vi "Launch Settings Dialog.vi"(8 "error in (no error)":errorcluster, 11 "Controller in":refnum<class "Controller.lvclass">) -> (0 "error out":errorcluster, 3 "Controller out":refnum<class "Controller.lvclass">)   [LabVIEW 2026, in "Controller Actor.lvlib" / "Controller.lvclass"]
uses:
  Controller.lvclass
  C:/Program Files/National Instruments/LabVIEW 2026/vi.lib/ActorFramework/Actor/Actor.lvclass
  Controller.lvclass/Controller.ctl
  <vilib>/ActorFramework/Actor/Actor.lvclass/Actor.ctl
  <vilib>/ActorFramework/Message Enqueuer/Message Enqueuer.lvclass/Message Enqueuer.ctl
  <vilib>/ActorFramework/Message Enqueuer/Init from Existing Queue.vi
  configuration/Configuration.lvclass
  <vilib>/ActorFramework/Message Enqueuer/Message Enqueuer.lvclass
  <vilib>/ActorFramework/Actor/Actor.lvclass
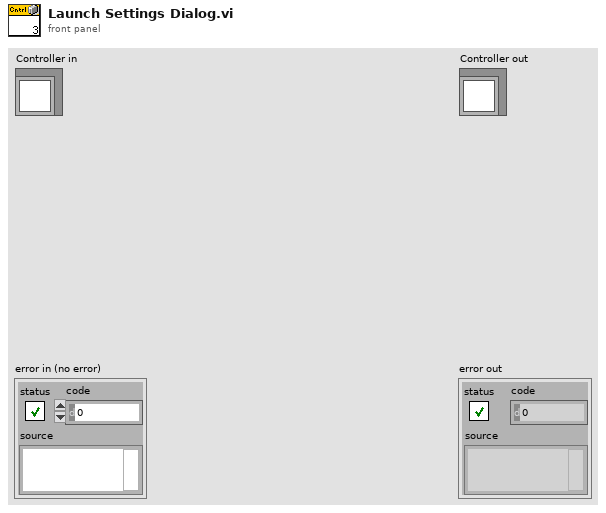
[diagram p1: front panel]
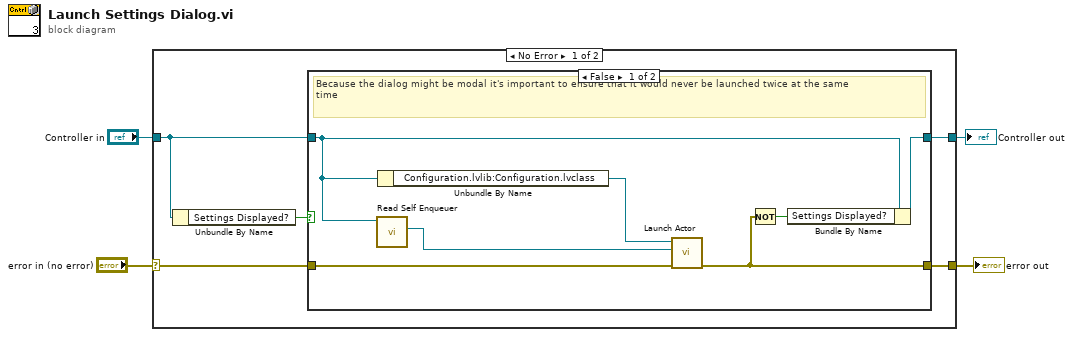
[diagram p0: block diagram]
diagram:
  n1 = case shown="No Error" "error in (no error)" {
    selector: "error in (no error)" -> [w5 w20]
    tunnel: [w8 w20] -> w3
    tunnel: [w9 w19] -> w1
    tunnel: "Controller in" -> [w7 w19]
    frame No Error {
      n2 = Unbundle By Name(w7) -> ("Settings Displayed?"=w6:bool)
      n3 = case shown="False" w6 {
        tunnel: [w14 w17] -> w9
        tunnel: [w12 w18] -> w8
        tunnel: w7 -> [w11 w17]
        tunnel: w5 -> [w10 w18]
        frame False {
          # "Because the dialog might be modal it's important to ensure that it would never be launched twice at the same\ntime"
          n4 = call <vilib>:"Read Self Enqueuer.vi"("Actor"=w11) -> ("Self Enqueuer"=w15:refnum<class "Message Enqueuer.lvclass">)  [unwired: 10 in]
          n5 = Unbundle By Name(w11) -> ("Configuration.lvlib:Configuration.lvclass"=w16:refnum<class "Configuration.lvclass">)
          n6 = call <vilib>:"Launch Actor.vi"("error in (no error)"=w10, "Actor-to-Caller Enqueuer"=w15, "Actor"=w16) -> ("error out"=w12:errorcluster)  [unwired: 7 in, 1 out]
          n7 = Not(x=w12) -> (.not. x?=w13:bool)
          n8 = Bundle By Name(cluster=w11, "Settings Displayed?"=w13) -> (w14:refnum<class "Controller.lvclass">)
        }
        frame True {
        }
      }
    }
    frame Error {
    }
  }
  "error out" <- w3
  "Controller out" <- w1
